vi "题目五.vi"() -> ()   [LabVIEW 2017]
panel:
  in  "数值":dbl
  out "通过":bool
  out "恭喜":bool
  out "警告":bool
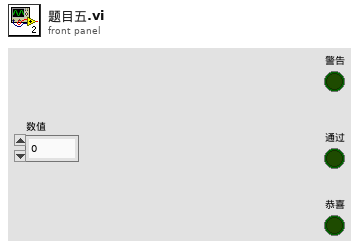
[diagram p1: front panel]
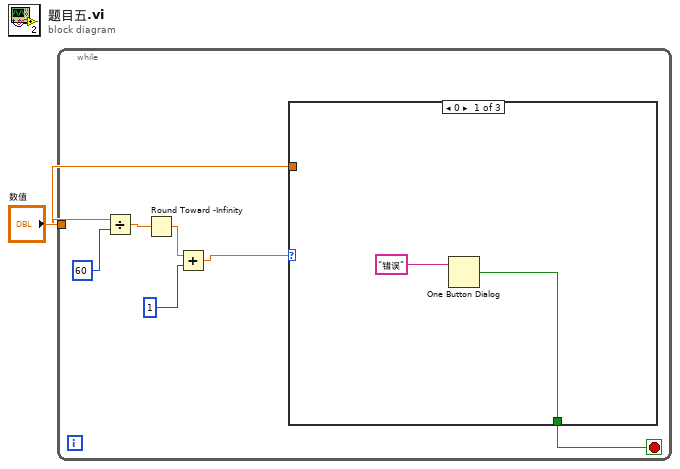
[diagram p0: block diagram]
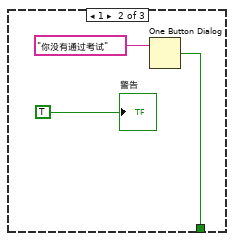
[diagram p2: hidden frame]
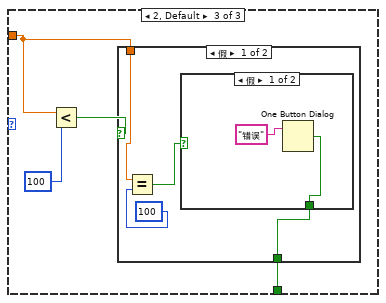
[diagram p3: hidden frame]
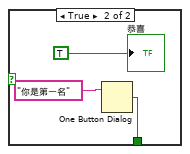
[diagram p4: hidden frame]
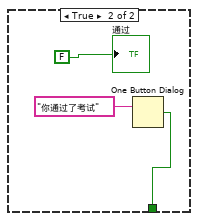
[diagram p5: hidden frame]
diagram:
  n1 = while {
    tunnel: "数值" -> [w2]
    stop <- w3 stop-if-true
    n2 = Divide(x=w2, y=60) -> (x/y=w7:dbl)
    n3 = Round Toward -Infinity(1:w7) -> (0:w5:dbl)
    n4 = Add(x=w5, y=1) -> (x+y=w4:dbl)
    n5 = case shown="0" w4 {
      tunnel: w2 -> [_ _ w14]
      tunnel: [w9 w11 w16] -> w3
      frame 0 {
        n6 = One Button Dialog(message="错误") -> (true=w9:bool)  [unwired: 1 in]
      }
      frame 1 {
        n7 = One Button Dialog(message="你没有通过考试") -> (true=w11:bool)  [unwired: 1 in]
        "警告" <- TRUE
      }
      frame 2, Default {
        n8 = Less?(x=w14, y=100) -> (x < y?=w15:bool)
        n9 = case shown="假" w15 {
          tunnel: [w21 w27] -> w16
          tunnel: w14 -> [w20 _]
          frame False {
            n10 = Equal?(x=w20, y=100) -> (x = y?=w18:bool)
            n11 = case shown="假" w18 {
              tunnel: [w22 w24] -> w21
              frame False {
                n12 = One Button Dialog(message="错误") -> (true=w22:bool)  [unwired: 1 in]
              }
              frame True {
                n13 = One Button Dialog(message="你是第一名") -> (true=w24:bool)  [unwired: 1 in]
                "恭喜" <- TRUE
              }
            }
          }
          frame True {
            n14 = One Button Dialog(message="你通过了考试") -> (true=w27:bool)  [unwired: 1 in]
            "通过" <- FALSE
          }
        }
      }
    }
  }
